vi "check for csv filename.vi"(9 "Canceled?":bool, 11 "selected path":path) -> (1 "file name":string, 2 "Result path":path, 3 "stripped path":path)   [LabVIEW 2016]
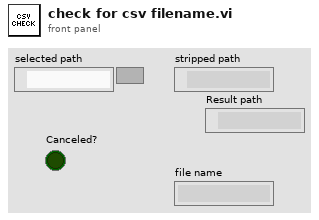
[diagram p1: front panel]
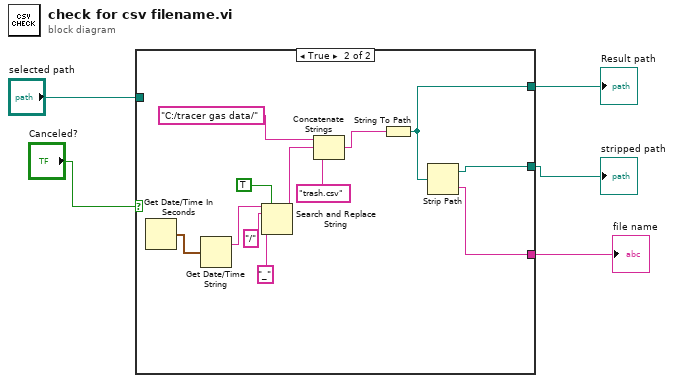
[diagram p0: block diagram]
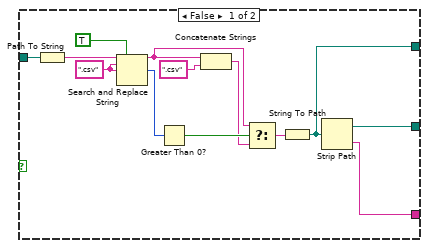
[diagram p2: hidden frame]
diagram:
  n1 = case shown="True" "Canceled?" {
    tunnel: "selected path" -> [w18 _]
    tunnel: [w8 w19] -> w4
    tunnel: [w7 w20] -> w3
    tunnel: [w6 w21] -> w2
    frame False {
      w9 = ".csv" ("replace string (\"\")")
      n2 = Path To String(path=w18) -> (string=w16:string)
      n3 = Search and Replace String(replace all?=TRUE ("replace all? (F)"), input string=w16, search string=w9, replace string=w9) -> (result string=w13:string, number of replacements=w14:i32)  [unwired: 4 in, 2 out]
      n4 = Greater Than 0?(x=w14) -> (x > 0?=w15:bool)
      n5 = Concatenate Strings(w13, ".csv" ("string")) -> (w12:string)
      n6 = Select(t=w13, s=w15, f=w12) -> (s? t:f=w11:string)
      n7 = String To Path(string=w11) -> (path=w6:path)
      n8 = Strip Path(path=w6) -> (stripped path=w7:path, name=w8:string)
    }
    frame True {
      n9 = Get Date/Time In Seconds() -> (seconds since 1Jan1904=w30:timestamp)
      n10 = Get Date/Time String(seconds (now)=w30) -> (date string=w27:string)  [unwired: 2 in, 1 out]
      n11 = Search and Replace String(replace all?=TRUE ("replace all? (F)"), input string=w27, search string="/", replace string="_" ("replace string (\"\")")) -> (result string=w28:string)  [unwired: 4 in, 3 out]
      n12 = Concatenate Strings("C:/tracer gas data/", w28, "trash.csv" ("string")) -> (w22:string)
      n13 = String To Path(string=w22) -> (path=w21:path)
      n14 = Strip Path(path=w21) -> (stripped path=w20:path, name=w19:string)
    }
  }
  "file name" <- w4
  "stripped path" <- w3
  "Result path" <- w2
